vi "Write RTDLRS1ADisplacementGauge.vi"(10 "RTDLRS1ADisplacementGauge.lvlib:DLRS1ADisplacementGauge.lvclass":refnum<class "DLRS1ADisplacementGauge.lvclass">, 11 "Model in":refnum<class "Model.lvclass">) -> (3 "Model out":refnum<class "Model.lvclass">)   [LabVIEW 2016, in "Model.lvclass"]
uses:
  Model.lvclass
  Common_RT_DLRS1ADisplacementGauge/DLRS1ADisplacementGauge/DLRS1ADisplacementGauge.lvclass
  Model.lvclass/Model.ctl
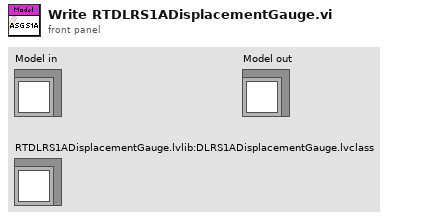
[diagram p1: front panel]
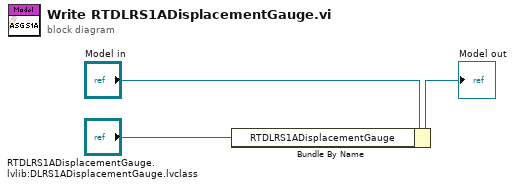
[diagram p0: block diagram]
diagram:
  n1 = Bundle By Name(cluster="Model in", "RTDLRS1ADisplacementGauge"="RTDLRS1ADisplacementGauge.lvlib:DLRS1ADisplacementGauge.lvclass") -> (→"Model out":refnum<class "Model.lvclass">)
